vi "I2C Write.vi"(0 "RedPitaya connection in":refnum<k5>, 3 "timeout ms (2000)":i32=2000, 5 "Address":u8 format="%x", 9 "Data":u8, 11 "error in":errorcluster) -> (4 "RedPitaya connection out":refnum<k5>, 15 "error out":errorcluster)   [LabVIEW 2021]
uses:
  Red_Pitaya_LabVIEW_Driver&Examples/Red_Pitaya/RedPitaya.lvlib
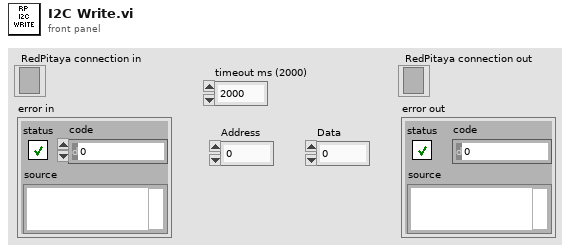
[diagram p1: front panel]
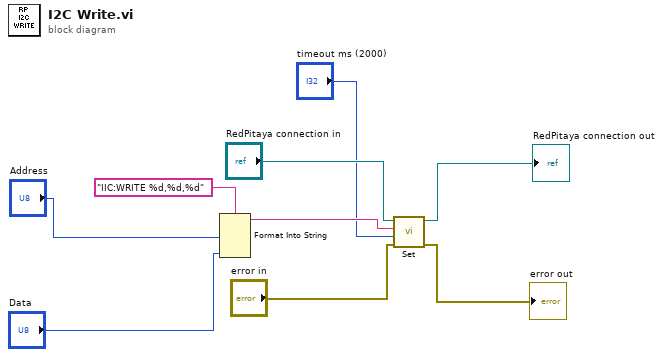
[diagram p0: block diagram]
diagram:
  n1 = Format Into String(format string="IIC:WRITE %d,%d,%d", "Address", "Data") -> (resulting string=w6:string, w3:u8)  [unwired: 2 in, 1 out]
  n2 = call "Set.vi"("error in"="error in", "timeout ms (2000)"="timeout ms (2000)", "SCPI Message"=w6, "RedPitaya connection in"="RedPitaya connection in") -> ("error out"=→"error out":errorcluster, "RedPitaya connection out"=→"RedPitaya connection out":refnum<k5>)  [unwired: 5 in, 1 out]
